vi "Configure Temperature Thermocouple.vi"(7 "Simulated Range":dbl, 8 "error in (no error)":errorcluster, 9 "Reference Junction":u16(ring) items=["Simulated", "Internal", "External"], 10 "Thermocouple Type":u16(ring) items=["B", "E", "J", "K", "N", "R", "S", "T"], 11 "VISA resource name":refnum<visa-resource-name>) -> (0 "error out":errorcluster, 3 "VISA resource name out":refnum<visa-resource-name>)   [LabVIEW 2009, in "Keithley DMM7510.lvlib"]
doc: "This VI configures the Temperature measurement function parameters like thermocouple type and related settings, reference junction type, simulated value."
uses:
  Keithley DMM7510.lvlib
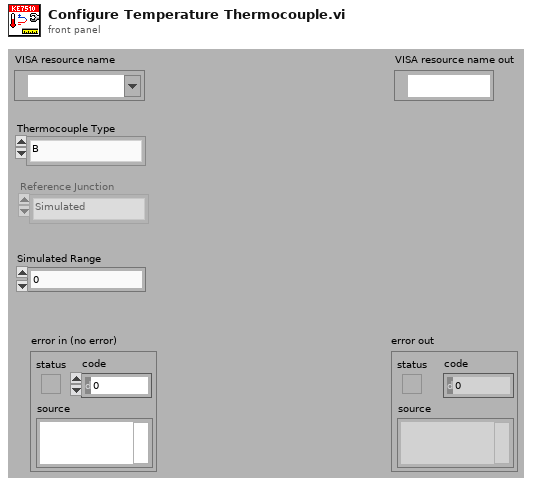
[diagram p1: front panel]
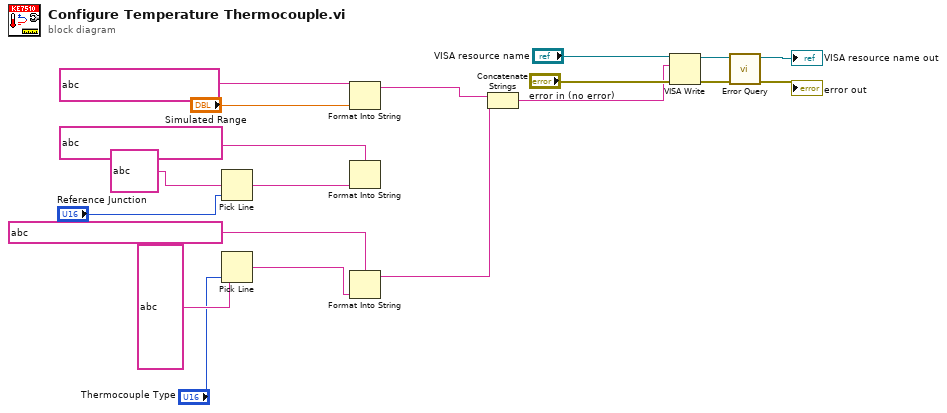
[diagram p0: block diagram]
diagram:
  n1 = Pick Line(multi-line string=string ?, line index="Reference Junction") -> (output string=w11:string)  [unwired: 1 in]
  n2 = Pick Line(multi-line string=string ?, line index="Thermocouple Type") -> (output string=w8:string)  [unwired: 1 in]
  n3 = Format Into String(format string=string ?, "Simulated Range") -> (resulting string=w14:string)  [unwired: 2 in, 1 out]
  n4 = Format Into String(format string=string ?, w11) -> ()  [unwired: 2 in, 2 out]
  n5 = Format Into String(format string=string ?, w8) -> (resulting string=w6:string)  [unwired: 2 in, 1 out]
  n6 = Concatenate Strings(w14, w6) -> (w13:string)
  n7 = VISA Write(VISA resource name="VISA resource name", write buffer=w13, error in (no error)="error in (no error)") -> (VISA resource name out=w5:refnum<visa-resource-name>, error out=w4:errorcluster)  [unwired: 1 out]
  n8 = call "Error Query.vi"("error in (no error)"=w4, "VISA resource name"=w5) -> ("error out"=→"error out":errorcluster, "VISA resource name out"=→"VISA resource name out":refnum<visa-resource-name>)  [unwired: 6 in, 2 out]
